vi "StartMeasurement.vi"(8 "error in (no error)":errorcluster, 11 "Actor in":refnum<class "Actor1_GUI_G4_4.0.0.lvclass">) -> (0 "error out":errorcluster, 3 "Actor out":refnum<class "Actor1_GUI_G4_4.0.0.lvclass">)   [LabVIEW 2020, in "Actor1_GUI_G4_4.0.0.lvlib" / "Actor1_GUI_G4_4.0.0.lvclass"]
uses:
  Actor1_GUI_G4_4.0.0.lvclass
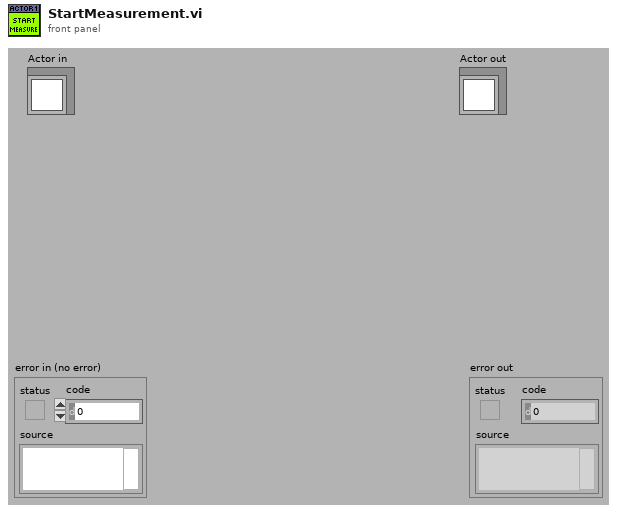
[diagram p1: front panel]
types:
  T1 = typedef "Actor1_GUI_G4_4.0.0.lvlib/Actor1_GUI_G4_4.0.0.lvclass/ObjectAttributes.ctl" = cluster{"LoopEvent":refnum<user-event>}
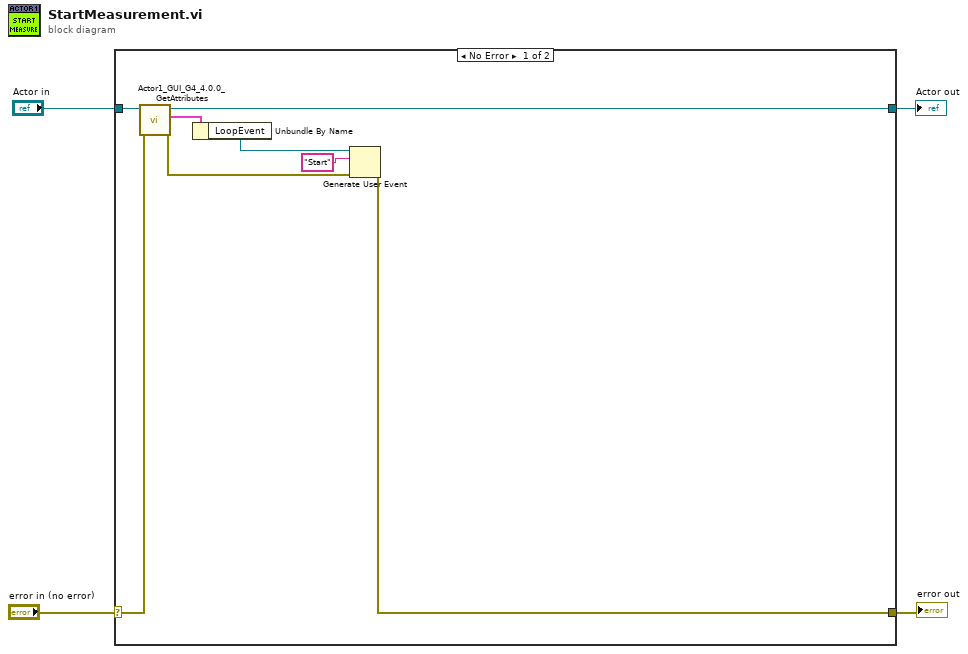
[diagram p0: block diagram]
diagram:
  n1 = case shown="No Error" "error in (no error)" {
    selector: "error in (no error)" -> [w9 w14]
    tunnel: [w12 w14] -> w3
    tunnel: [w10 w13] -> w1
    tunnel: "Actor in" -> [w11 w13]
    frame No Error {
      n2 = call "Actor1_GUI_G4_4.0.0_GetAttributes.vi"("error in (no error)"=w9, "reference in"=w11) -> ("error out"=w8:errorcluster, "Data"=w7:T1, "reference out"=w10:refnum<class "Actor1_GUI_G4_4.0.0.lvclass">)  [unwired: 6 in, 1 out]
      n3 = Unbundle By Name(w7) -> ("LoopEvent"=w6:refnum<user-event>)
      n4 = Generate User Event(user event=w6, event data cluster="Start" ("event data"), error in=w8) -> (error out=w12:errorcluster)  [unwired: 1 in, 1 out]
    }
    frame Error {
    }
  }
  "error out" <- w3
  "Actor out" <- w1
